vi "get values from html (SubVI).vi"(10 "Sensor URL":string, 11 "Cluster in":T1) -> (3 "Cluster out":T1)   [LabVIEW 2013]
uses:
  <vilib>/regexp/Match Regular Expression.xnode
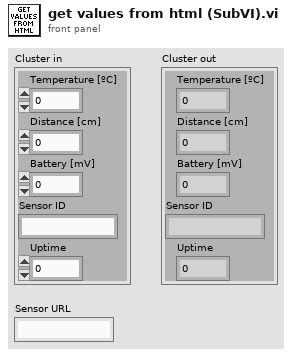
[diagram p1: front panel]
types:
  T1 = cluster{"Temperature [ºC] ":dbl, "Distance [cm]":dbl, "Battery [mV]":dbl, "Sensor ID":string, "Uptime":dbl}
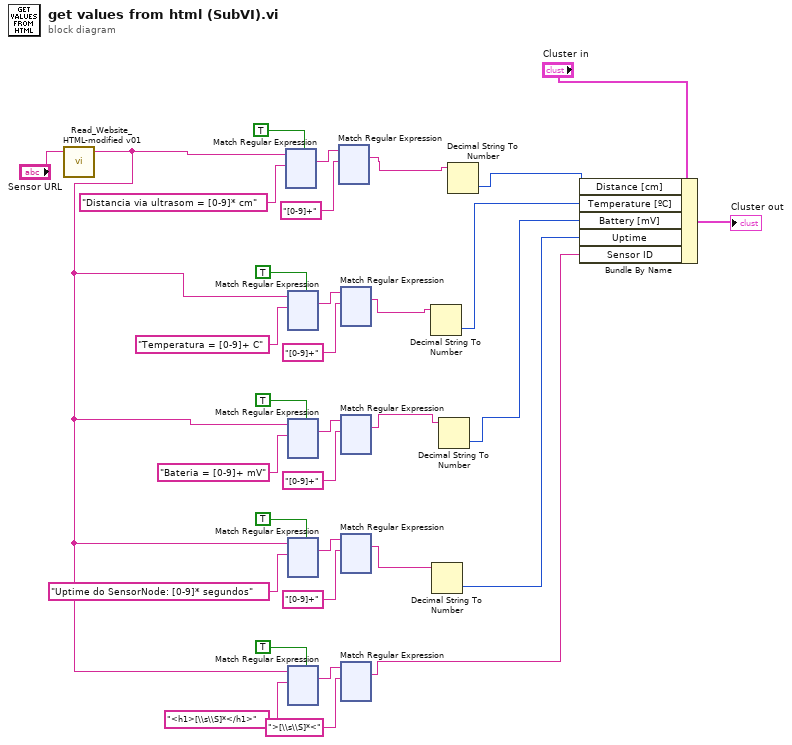
[diagram p0: block diagram]
diagram:
  n1 = call "Read_Website_HTML-modified v01.vi"("URL"="Sensor URL") -> ("HTML as string"=w23:string)  [unwired: 3 in, 1 out]
  n2 = xnode "Match Regular Expression"("input string"=w23, "regular expression"="Distancia via ultrasom = [0-9]* cm", "multiline? (F)"=TRUE) -> ("whole match"=w3:string)  [unwired: 3 in, 4 out]
  n3 = xnode "Match Regular Expression"("input string"=w23, "regular expression"="Temperatura = [0-9]+ C", "multiline? (F)"=TRUE) -> ("whole match"=w7:string)  [unwired: 3 in, 4 out]
  n4 = xnode "Match Regular Expression"("input string"=w23, "regular expression"="Bateria = [0-9]+ mV", "multiline? (F)"=TRUE) -> ("whole match"=w11:string)  [unwired: 3 in, 4 out]
  n5 = xnode "Match Regular Expression"("input string"=w23, "regular expression"="Uptime do SensorNode: [0-9]* segundos", "multiline? (F)"=TRUE) -> ("whole match"=w15:string)  [unwired: 3 in, 4 out]
  n6 = xnode "Match Regular Expression"("input string"=w23, "regular expression"="<h1>[\\s\\S]*</h1>", "multiline? (F)"=TRUE) -> ("whole match"=w19:string)  [unwired: 3 in, 4 out]
  n7 = xnode "Match Regular Expression"("input string"=w3, "regular expression"="[0-9]+") -> ("whole match"=w22:string)  [unwired: 4 in, 4 out]
  n8 = xnode "Match Regular Expression"("input string"=w7, "regular expression"="[0-9]+") -> ("whole match"=w24:string)  [unwired: 4 in, 4 out]
  n9 = xnode "Match Regular Expression"("input string"=w11, "regular expression"="[0-9]+") -> ("whole match"=w25:string)  [unwired: 4 in, 4 out]
  n10 = xnode "Match Regular Expression"("input string"=w15, "regular expression"="[0-9]+") -> ("whole match"=w26:string)  [unwired: 4 in, 4 out]
  n11 = xnode "Match Regular Expression"("input string"=w19, "regular expression"=">[\\s\\S]*<") -> ("whole match"=w32:string)  [unwired: 4 in, 4 out]
  n12 = Decimal String To Number(string=w24) -> (number=w29:i32)  [unwired: 2 in, 1 out]
  n13 = Decimal String To Number(string=w26) -> (number=w31:i32)  [unwired: 2 in, 1 out]
  n14 = Decimal String To Number(string=w25) -> (number=w30:i32)  [unwired: 2 in, 1 out]
  n15 = Decimal String To Number(string=w22) -> (number=w28:i32)  [unwired: 2 in, 1 out]
  n16 = Bundle By Name(cluster="Cluster in", "Distance [cm]"=w28, "Temperature [ºC]"=w29, "Battery [mV]"=w30, "Uptime"=w31, "Sensor ID"=w32) -> (→"Cluster out":T1)
